vi "IFD Tag to File.vi"(8 "error in (no error)":errorcluster, 9 "Last Reference Offset":u32, 10 "refnum in":refnum<file>, 11 "IFD in":refnum<class "IFD.lvclass">) -> (0 "error out":errorcluster, 1 "Reference Offset":u32, 2 "refnum out":refnum<file>, 3 "IFD out":refnum<class "IFD.lvclass">)   [LabVIEW 2016, in "IFD.lvclass"]
uses:
  IFD.lvclass
  IFD.lvclass/IFD.ctl
  Tag/IFD_Tag.lvclass
  Tag/Offset Content.ctl
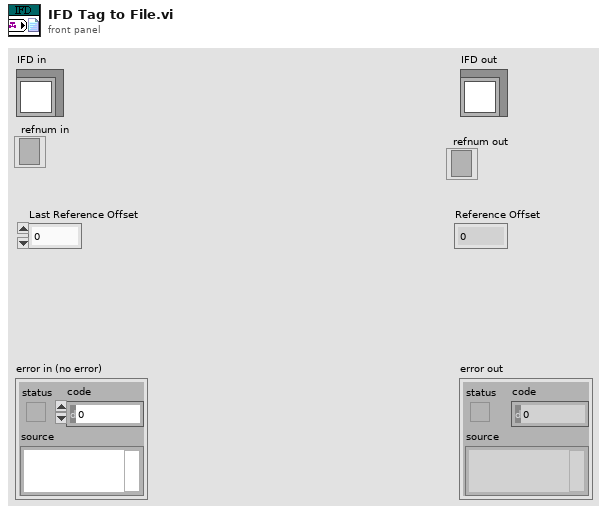
[diagram p1: front panel]
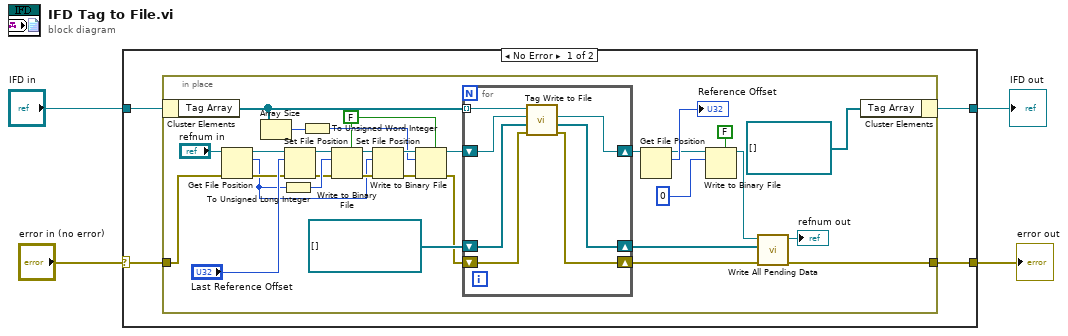
[diagram p0: block diagram]
diagram:
  n1 = case shown="No Error" "error in (no error)" {
    selector: "error in (no error)" -> [w6 w48]
    tunnel: [w5 w48] -> w3
    tunnel: [w7 w47] -> w1
    tunnel: "IFD in" -> [w8 w47]
    frame No Error {
      n2 = in-place {
        in-place-border: w6 -> [w15]
        in-place-border: [w34] -> w5
        w18 = FALSE ("prepend array or string size? (T)")
        n3 = in-place-cluster #1(w8) -> ("Tag Array"=w33:refnum<class "IFD_Tag.lvclass">[])
        n4 = Get File Position(4:w15, 7:"refnum in") -> (0:w14:errorcluster, 2:w9:i64, 3:w31:refnum<file>)
        n5 = Array Size(array=w33) -> (size(s)=w25:i32)
        n6 = To Unsigned Long Integer(number=w9) -> (unsigned 32bit integer=w27:u32)
        n7 = Set File Position(offset (in bytes) (0)="Last Reference Offset", refnum=w31, error in=w14) -> (refnum out=w29:refnum<file>, error out=w13:errorcluster)  [unwired: 1 in]
        n8 = To Unsigned Word Integer(number=w25) -> (unsigned 16bit integer=w24:u16)
        n9 = Write to Binary File(file (use dialog)=w29, data=w27, error in=w13, 5:w18) -> (refnum out=w28:refnum<file>, error out=w12:errorcluster)  [unwired: 2 in, 1 out]
        n10 = Set File Position(offset (in bytes) (0)=w9, refnum=w28, error in=w12) -> (refnum out=w26:refnum<file>, error out=w11:errorcluster)  [unwired: 1 in]
        n11 = Write to Binary File(file (use dialog)=w26, data=w24, error in=w11, 5:w18) -> (refnum out=w23:refnum<file>, error out=w10:errorcluster)  [unwired: 2 in, 1 out]
        n12 = for {
          tunnel: w33 -> [w46] mode=indexing
          shift-right: [w44] -> w22
          shift-left: w23 -> [w45]
          shift-right: [w42] -> w37
          shift-left: refnum<data-value>[] [] ("Pending data in") -> [w43]
          shift-right: [w40] -> w36
          shift-left: w10 -> [w41]
          n13 = call "Tag Write to File.vi"("error in (no error)"=w41, "Pending data in"=w43, "refnum in"=w45, "IFD_Tag in"=w46) -> ("error out"=w40:errorcluster, "Pending data out"=w42:refnum<data-value>[], "refnum out"=w44:refnum<file>)  [unwired: 5 in]
        }
        n14 = Get File Position(7:w22) -> (2:→"Reference Offset":i64, 3:w20:refnum<file>)  [unwired: 1 in, 1 out]
        n15 = Write to Binary File(file (use dialog)=w20, data=u32 0, 5:FALSE ("prepend array or string size? (T)")) -> (refnum out=w16:refnum<file>)  [unwired: 3 in, 2 out]
        n16 = call "Write All Pending Data.vi"("error in (no error)"=w36, "Pending data"=w37, "refnum in"=w16) -> ("error out"=w34:errorcluster, "refnum out"=→"refnum out":refnum<file>)  [unwired: 7 in]
        n17 = in-place-cluster #1("Tag Array"=refnum<class "IFD_Tag.lvclass">[] []) -> (w7:refnum<class "IFD.lvclass">)
      }
    }
    frame Error {
    }
  }
  "error out" <- w3
  "IFD out" <- w1
